vi "Renju.vi"() -> ()   [LabVIEW 2015]
uses:
  Controls/Chess Control.ctl
  <vilib>/Utility/miscctls.llb/LVPointTypeDef.ctl
panel:
  in  "Detect":bool[][](array[boolean])=[[FALSE, FALSE, FALSE, FALSE, FALSE, FALSE, FALSE, FALSE, FALSE, FALSE], [FALSE, FALSE, FALSE, FALSE, FALSE, FALSE, FALSE, FALSE, FALSE, FALSE], [FALSE, FALSE, FALSE, FALSE, FALSE, FALSE, FALSE, FALSE, FALSE, FALSE], [FALSE, FALSE, FALSE, FALSE, FALSE, FALSE, FALSE, FALSE, FALSE, FALSE], [FALSE, FALSE, FALSE, FALSE, FALSE, FALSE, FALSE, FALSE, FALSE, FALSE], [FALSE, FALSE, FALSE, FALSE, FALSE, FALSE, FALSE, FALSE, FALSE, FALSE], [FALSE, FALSE, FALSE, FALSE, FALSE, FALSE, FALSE, FALSE, FALSE, FALSE], [FALSE, FALSE, FALSE, FALSE, FALSE, FALSE, FALSE, FALSE, FALSE, FALSE], [FALSE, FALSE, FALSE, FALSE, FALSE, FALSE, FALSE, FALSE, FALSE, FALSE], [FALSE, FALSE, FALSE, FALSE, FALSE, FALSE, FALSE, FALSE, FALSE, FALSE]]
  out "ChessBoard":T1[][](array[typedef])
  in  "Restart":bool
  in  "Stop":bool
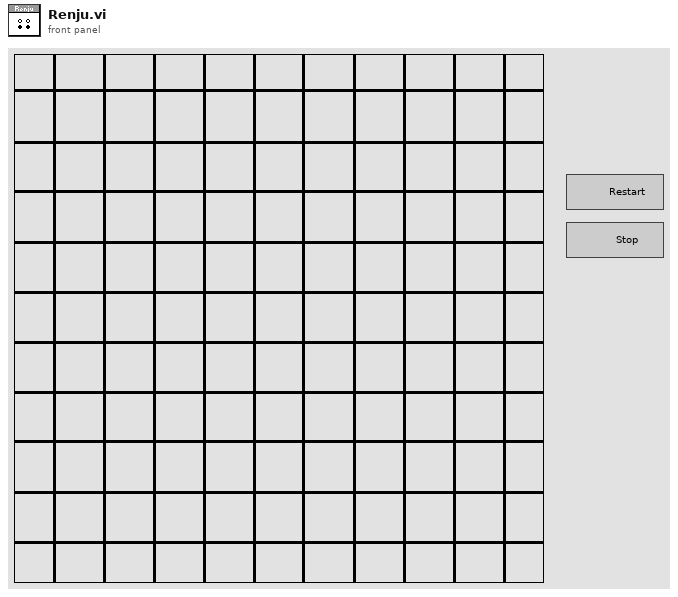
[diagram p1: front panel]
types:
  T1 = typedef "Chess Control.ctl" = u16
  T2 = typedef "LVPointTypeDef.ctl" = cluster{"Horizontal":i16, "Vertical":i16}
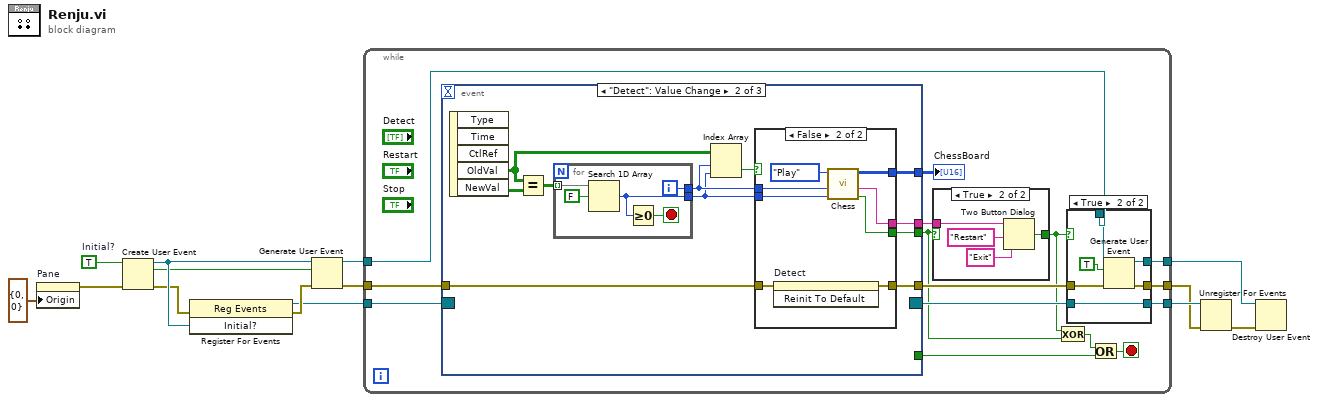
[diagram p0: block diagram]
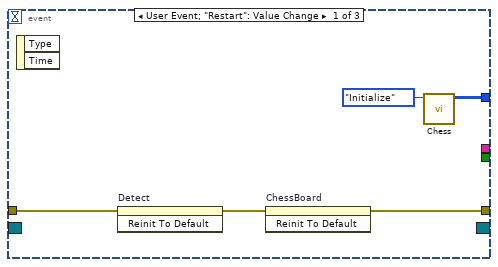
[diagram p4: hidden frame]
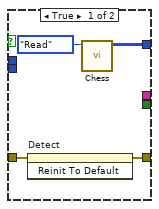
[diagram p5: hidden frame]
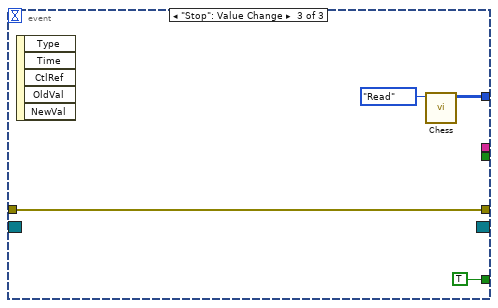
[diagram p6: hidden frame]
diagram:
  w7 = TRUE  # Initial?
  n1 = property on="Pane" class="Pane"("Origin"=T2 {"Horizontal"=0, "Vertical"=0}) -> (error out=w1:errorcluster)  [unwired: 2 in, 1 out]
  n2 = Create User Event(user event datatype=w7, error in=w1) -> (user event=w13:refnum<user-event>, error out=w12:errorcluster)
  n3 = register-events(error in=w12, w13) -> (reference out=w10:refnum<event-registration>, error out=w11:errorcluster)  [unwired: 1 in]
  n4 = Generate User Event(user event=w13, event data cluster=w7, error in=w11) -> (user event out=w9:refnum<user-event>, error out=w8:errorcluster)  [unwired: 1 in]
  n5 = while {
    tunnel: w10 -> [w28]
    tunnel: w9 -> [w21]
    tunnel: w8 -> [w27]
    tunnel: [w22] -> w6
    tunnel: [w24] -> w5
    tunnel: [w20] -> w3
    stop <- w14 stop-if-true
    n6 = event shown="[1] \"Detect\": Value Change" {
      selector: w28 -> [_ _ _]
      dyn-events: [_ _ _] -> w23
      timeout: _ -> [_ _ _]
      tunnel: w27 -> [w46 w51 w77]
      tunnel: [w44 w50 w77] -> w25
      tunnel: [w43 w49 w76] -> w26
      tunnel: [_ _ TRUE] -> w15
      tunnel: [_ w48 _] -> w18
      tunnel: [_ w47 _] -> w17
      event User Event; "Restart": Value Change {
        n7 = event-data() -> ()  [unwired: 1 in, 2 out]
        n8 = invoke on="Detect" class="Arr (strict)" method="Reinit To Default"(error in=w46) -> (error out=w45:errorcluster)  [unwired: 2 in, 2 out]
        n9 = invoke on="ChessBoard" class="Arr (strict)" method="Reinit To Default"(error in=w45) -> (error out=w44:errorcluster)  [unwired: 2 in, 2 out]
        n10 = call "Chess.vi"("State"=enum16{"Initialize", "Play", "Read"}."Initialize") -> ("Data"=w43:u16[][])  [unwired: 8 in, 2 out]
      }
      event "Detect": Value Change {
        n11 = event-data() -> ("OldVal"=w55:bool[][], "NewVal"=w56:bool[][])  [unwired: 1 in, 3 out]
        n12 = Equal?(x=w55, y=w56) -> (x = y?=w57:bool[][])
        n13 = for {
          tunnel: w57 -> [w74] mode=indexing
          tunnel: [w72] -> w53
          tunnel: [w71] -> w54
          i -> [w71]
          stop <- w70 stop-if-true
          n14 = Search 1D Array(1D array=w74, element=FALSE) -> (index of element=w72:i32)  [unwired: 1 in]
          n15 = Greater Or Equal To 0?(x=w72) -> (x >= 0?=w70:bool)
        }
        n16 = Index Array(array=w55, index (row)=w54, index (col)=w53) -> (element=w52:bool)
        n17 = case shown="False" w52 {
          tunnel: w54 -> [_ w67]
          tunnel: w53 -> [_ w66]
          tunnel: w51 -> [w61 w69]
          tunnel: [w60 w68] -> w50
          tunnel: [w58 w64] -> w49
          tunnel: [_ w62] -> w48
          tunnel: [_ w63] -> w47
          frame True {
            n18 = invoke on="Detect" class="Arr (strict)" method="Reinit To Default"(error in=w61) -> (error out=w60:errorcluster)  [unwired: 2 in, 2 out]
            n19 = call "Chess.vi"("State"=enum16{"Initialize", "Play", "Read"}."Read") -> ("Data"=w58:u16[][])  [unwired: 8 in, 2 out]
          }
          frame False {
            n20 = invoke on="Detect" class="Arr (strict)" method="Reinit To Default"(error in=w69) -> (error out=w68:errorcluster)  [unwired: 2 in, 2 out]
            n21 = call "Chess.vi"("column"=w66, "row"=w67, "State"=enum16{"Initialize", "Play", "Read"}."Play") -> ("Over?"=w63:bool, "Message"=w62:string, "Data"=w64:u16[][])  [unwired: 6 in]
          }
        }
      }
      event "Stop": Value Change {
        n22 = event-data() -> ()  [unwired: 1 in, 5 out]
        n23 = call "Chess.vi"("State"=enum16{"Initialize", "Play", "Read"}."Read") -> ("Data"=w76:u16[][])  [unwired: 8 in, 2 out]
      }
    }
    "ChessBoard" <- w26
    n24 = case shown="True" w17 {
      tunnel: [_ w30] -> w19
      tunnel: w18 -> [_ w29]
      frame False {
      }
      frame True {
        n25 = Two Button Dialog(message=w29, 1:"Exit" ("F button name (\"Cancel\")"), 2:"Restart" ("T button name (\"OK\")")) -> (T button?=w30:bool)
      }
    }
    n26 = Exclusive Or(1:w17, 2:w19) -> (0:w16:bool)
    n27 = case shown="True" w19 {
      tunnel: w25 -> [w34 w41]
      tunnel: [w34 w40] -> w24
      tunnel: w23 -> [w35 w39]
      tunnel: [w35 w39] -> w22
      tunnel: w21 -> [w33 w38]
      tunnel: [w33 w37] -> w20
      frame False {
      }
      frame True {
        n28 = Generate User Event(user event=w38, event data cluster=TRUE ("event data"), error in=w41) -> (user event out=w37:refnum<user-event>, error out=w40:errorcluster)  [unwired: 1 in]
      }
    }
    n29 = Or(x=w16, y=w15) -> (x .or. y?=w14:bool)
  }
  n30 = Unregister For Events(event registration refnum=w6, error in=w5) -> (error out=w4:errorcluster)
  n31 = Destroy User Event(user event=w3, error in=w4) -> ()  [unwired: 1 out]
